vi "Intake Globals.vi"() -> ()   [LabVIEW 2017]
uses:
  Intake Notifier.ctl
  Intake Control Type.ctl
panel:
  out "Cube IR":bool
  in  "Intake Cals":dbl[](array[numeric])
  in  "Intake Execute Notifier":refnum<notifier>
  in  "Intake Set Notifier":refnum<notifier>
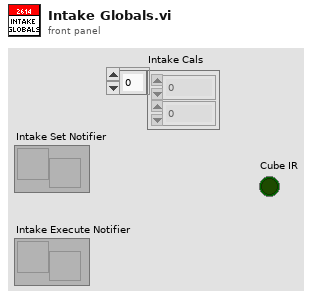
[diagram p1: front panel]
diagram:
